vi "Instrument Info.vi"(8 "error in (no error)":errorcluster, 11 "VISA resource name":refnum<visa-resource-name>) -> (0 "error out":errorcluster, 2 "Instr Model":u32, 3 "VISA resource name out":refnum<visa-resource-name>, 5 "Channels":i32)   [LabVIEW 2012, in "Berkeley Nucleonics 500 Series.lvlib"]
doc: "This utility VI returns the option number, model number, and number of channels of the unit."
uses:
  Berkeley Nucleonics 500 Series.lvlib
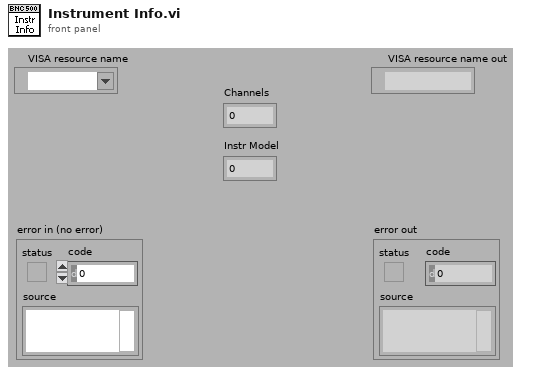
[diagram p1: front panel]
types:
  T1 = enum16{"Read Data", "Write Data", "Dispose of Data", "Clear ALL Data"}
  T2 = typedef "Berkeley Nucleonics 500 Series.lvlib/Unit Info.ctl" = cluster{"ID String":string, "Model":string, "Model #":i32, "# Channels":i32, "Options":string, "Firmware":string, "FPGA Ver":string}
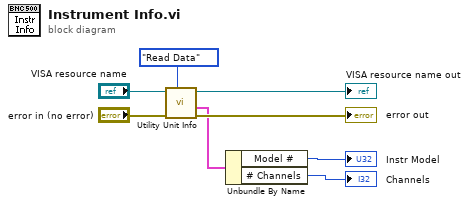
[diagram p0: block diagram]
diagram:
  n1 = call "Utility Unit Info.vi"("Action"=T1."Read Data", "Error In (no error)"="error in (no error)", "VISA resource name in"="VISA resource name") -> ("Error Out"=→"error out":errorcluster, "Unit Info Out"=w3:T2, "VISA resource name out"=→"VISA resource name out":refnum<visa-resource-name>)  [unwired: 1 in, 5 out]
  n2 = Unbundle By Name(w3) -> ("Model #"=→"Instr Model":i32, "# Channels"=→"Channels":i32)
